vi "Enable_Signal_WPC.vi"(8 "error in (no error)":errorcluster, 10 "Enable (active low)":bool) -> (0 "error out":errorcluster)   [LabVIEW 2014]
uses:
  Functional_Global/Typedef_FPGA_Interface_Action.ctl
  <vilib>/Utility/error.llb/Error Cluster From Error Code.vi
  <vilib>/rvi/errors/niLvFpgaAdjustHostInterfaceError.vi
  <vilib>/rvi/interface/nirviReadWriteControl/nirviReadWriteControl.xnode
  NiFpgaLv.dll
  <vilib>/rvi/interface/Simulation/niFpgaSimulationCallBeginRW.vi
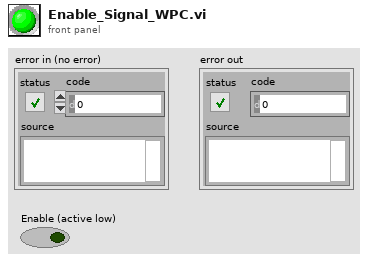
[diagram p1: front panel]
types:
  T1 = typedef "Typedef_FPGA_Interface_Action.ctl" = enum16{"Initialize FPGA", "Get FPGA Reference", "Close FPGA"}
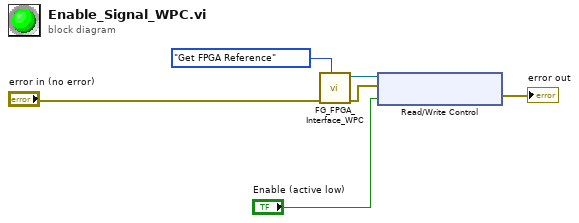
[diagram p0: block diagram]
diagram:
  n1 = call "FG_FPGA_Interface_WPC.vi"("Action"=Typedef_FPGA_Interface_Action."Get FPGA Reference", "error in"="error in (no error)") -> ("error out"=w5:errorcluster, "FPGA VI Reference Out"=w4:refnum<k20>)  [unwired: 8 in]
  n2 = xnode "Read/Write Control"("FPGA VI Reference In"=w4, "error in"=w5, "Enable (active low)"="Enable (active low)") -> ("error out"=→"error out":errorcluster)  [unwired: 1 out]
